vi "EnumerateDataTypes.vi"(8 "error in (no error)":errorcluster, 11 "Web Service Importer in":refnum<k24>) -> (0 "error out":errorcluster, 2 "Data Types":string[](array[string]), 3 "Web Service Importer out":refnum<k24>)   [LabVIEW 2017]
uses:
  e:/builds/penguin/labview/branches/2017/dev/dist/resource/WebServiceUtils.dll
  resource/WebServiceUtils.dll
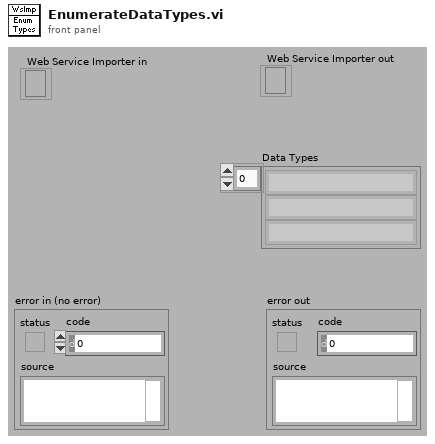
[diagram p1: front panel]
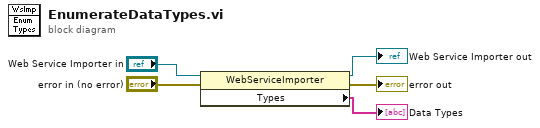
[diagram p0: block diagram]
diagram:
  n1 = property class="WebServiceImporter"(reference="Web Service Importer in", error in="error in (no error)") -> (reference out=→"Web Service Importer out":refnum<k24>, error out=→"error out":errorcluster, "Types"=→"Data Types":string[])
